vi "Star_buzz_main.vi"() -> ()   [LabVIEW 2019]
uses:
  Beverage/Espresso/Espresso.lvclass
  D:/LabVIEW/LabVIEW codes/solutions_and_repetitions/Decorator_pattern/Beverage/Beverage.lvclass
  Beverage/Dark Roast/Dark Roast.lvclass
  Beverage/Condiment Decorator/Milk/Milk.lvclass
  Beverage/Condiment Decorator/Mocha/Mocha.lvclass
  Beverage/House Blend/House Blend.lvclass
  Beverage/Condiment Decorator/Soy/Soy.lvclass
  Beverage/Condiment Decorator/Whip/Whip.lvclass
  Beverage/Beverage.lvclass
panel:
  out "Your Order":string
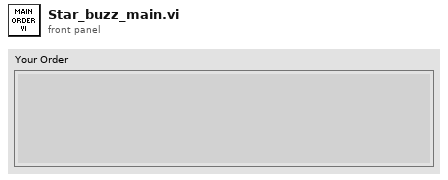
[diagram p1: front panel]
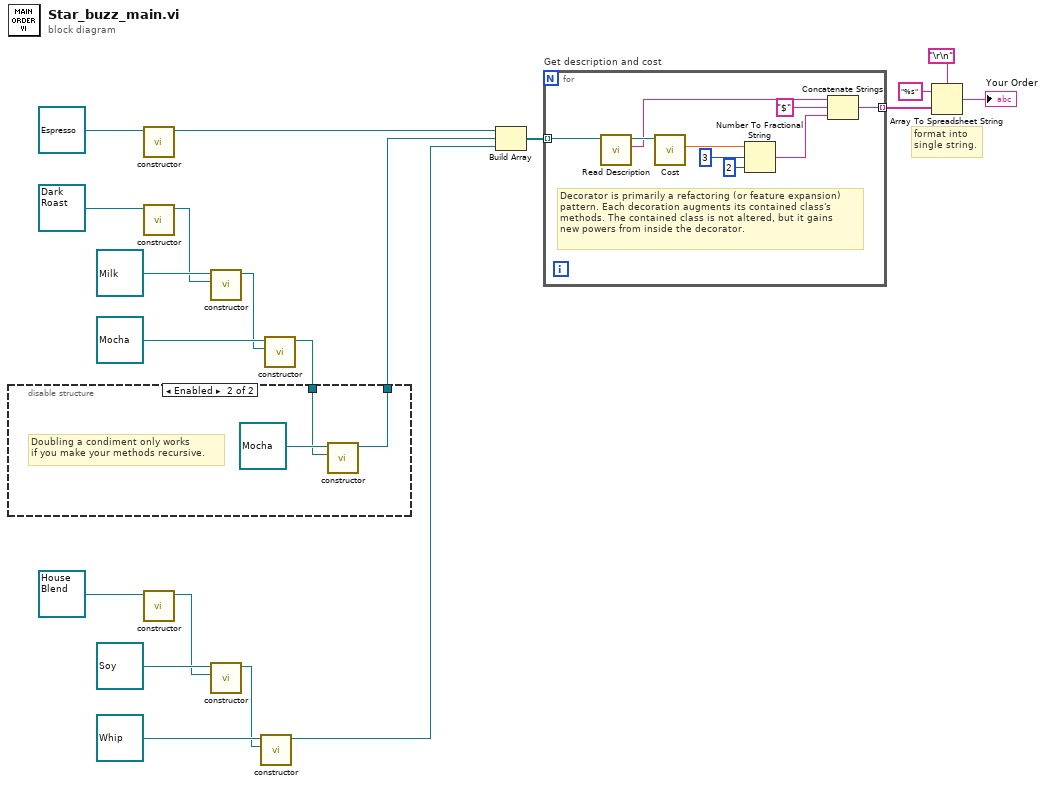
[diagram p0: block diagram]
diagram:
  # "format into\nsingle string."
  n1 = call-dynamic "constructor.vi"("Espresso in"=refnum<class "Espresso.lvclass"> refnum ("Espresso.lvclass")) -> ("Espresso out"=w19:refnum<class "Espresso.lvclass">)  [unwired: 10 in]
  n2 = call-dynamic "constructor.vi"("Dark Roast in"=refnum<class "Dark Roast.lvclass"> refnum ("Dark Roast.lvclass")) -> ("Dark Roast out"=w16:refnum<class "Dark Roast.lvclass">)  [unwired: 10 in]
  n3 = call-dynamic "constructor.vi"("House Blend in"=refnum<class "House Blend.lvclass"> refnum ("House Blend.lvclass")) -> ("House Blend out"=w9:refnum<class "House Blend.lvclass">)  [unwired: 10 in]
  n4 = call-dynamic "constructor.vi"("Beverage.lvclass"=w16, "Milk in"=refnum<class "Milk.lvclass"> refnum ("Milk.lvclass")) -> ("Milk out"=w14:refnum<class "Milk.lvclass">)  [unwired: 9 in]
  n5 = call-dynamic "constructor.vi"("Beverage.lvclass"=w9, "Soy in"=refnum<class "Soy.lvclass"> refnum ("Soy.lvclass")) -> ("Soy out"=w7:refnum<class "Soy.lvclass">)  [unwired: 9 in]
  n6 = call-dynamic "constructor.vi"("Beverage.lvclass"=w7, "Whip in"=refnum<class "Whip.lvclass"> refnum ("Whip.lvclass")) -> ("Whip out"=w6:refnum<class "Whip.lvclass">)  [unwired: 9 in]
  n7 = call-dynamic "constructor.vi"("Beverage.lvclass"=w14, "Mocha in"=refnum<class "Mocha.lvclass"> refnum ("Mocha.lvclass")) -> ("Mocha out"=w13:refnum<class "Mocha.lvclass">)  [unwired: 9 in]
  n8 = disable-structure shown="Enabled" {
    disable-tunnel: w13 -> [w21 w23]
    disable-tunnel: [w21 w22] -> w12
    frame Disabled {
    }
    frame Enabled {
      # "Doubling a condiment only works\nif you make your methods recursive."
      n9 = call-dynamic "constructor.vi"("Beverage.lvclass"=w23, "Mocha in"=refnum<class "Mocha.lvclass"> refnum ("Mocha.lvclass")) -> ("Mocha out"=w22:refnum<class "Mocha.lvclass">)  [unwired: 9 in]
    }
  }
  n10 = Build Array(w19, w12, w6) -> (w5:refnum<class "Beverage.lvclass">[])
  n11 = for "Get description and cost" {
    tunnel: w5 -> [w33] mode=indexing
    tunnel: [w25] -> w4 mode=indexing
    # "Decorator is primarily a refactoring (or feature expansion)\npattern. Each decoration augments its contained class's\nmethods. The contained class is not altered, but it gains\nnew powers from inside the decorator."
    n12 = call-dynamic "Read Description.vi"("Beverage in"=w33) -> ("Description"=w28:string, "Beverage out"=w32:refnum<class "Beverage.lvclass">)  [unwired: 9 in]
    n13 = call-dynamic "Cost.vi"("Beverage in"=w32) -> ("Cost"=w31:dbl)  [unwired: 8 in, 2 out]
    n14 = Number To Fractional String(number=w31, width (-)=i16 3, precision (6)=i16 2) -> (F-format string=w26:string)  [unwired: 1 in]
    n15 = Concatenate Strings(w28, "$" ("string"), w26) -> (w25:string)
  }
  n16 = Array To Spreadsheet String(delimiter (Tab)="\r\n", array=w4, 3:"%s" ("format string")) -> (spreadsheet string=→"Your Order":string)
